vi "Find Supported By.vi"(11 "Bricks in":T1(array[cluster])) -> (3 "Bricks out":T1(array[cluster]))   [LabVIEW 2023, in "d22.lvlib"]
uses:
  d22.lvlib
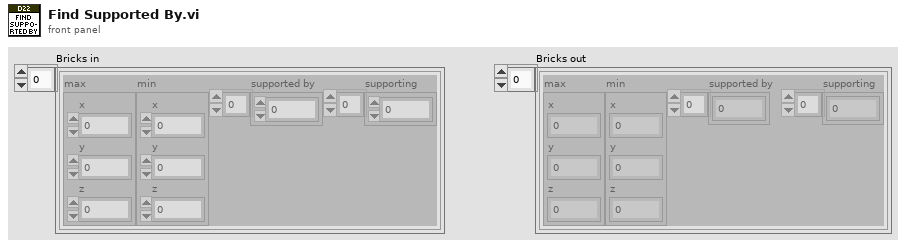
[diagram p1: front panel]
types:
  T1 = cluster{"max":cluster{"x":i32, "y":i32, "z":i32}, "min":cluster{"x":i32, "y":i32, "z":i32}, "supported by":i32[], "supporting":i32[]}[]
  T2 = cluster{"max":cluster{"x":i32, "y":i32, "z":i32}, "min":cluster{"x":i32, "y":i32, "z":i32}, "supported by":i32[], "supporting":i32[]}
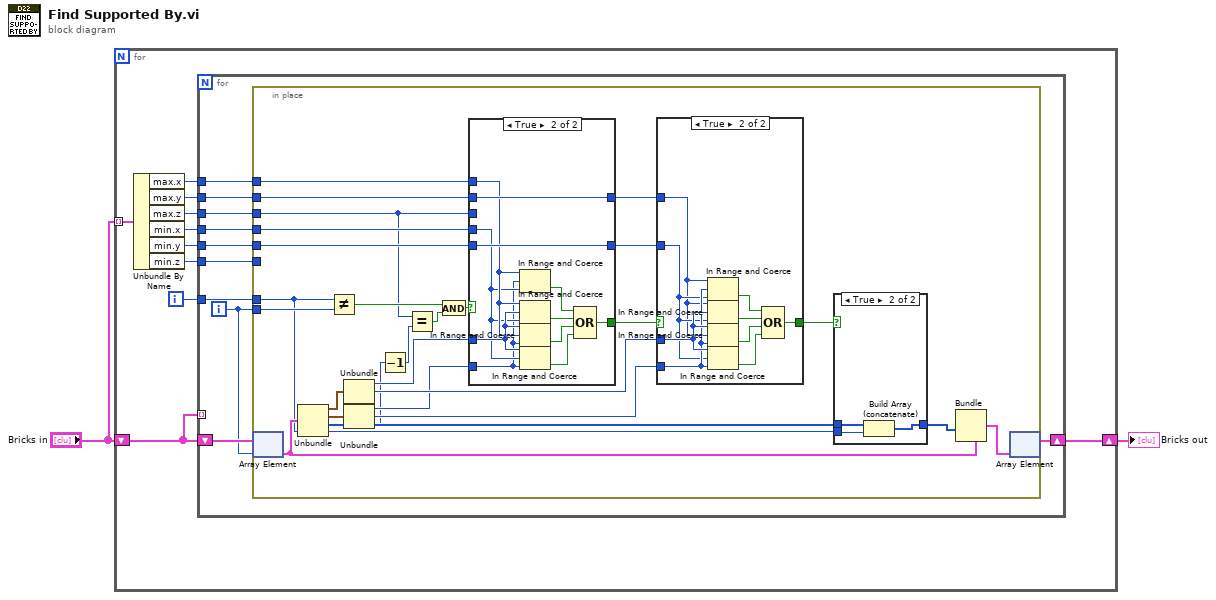
[diagram p0: block diagram]
diagram:
  n1 = for {
    shift-right: [w11] -> w2
    shift-left: "Bricks in" -> [w3]
    tunnel: "Bricks in" -> [w10] mode=indexing
    i -> [w12]
    n2 = Unbundle By Name(w10) -> ("max.x"=w8:i32, "max.y"=w9:i32, "max.z"=w7:i32, "min.x"=w6:i32, "min.y"=w5:i32, "min.z"=w4:i32)
    n3 = for {
      tunnel: w9 -> [w21]
      tunnel: w8 -> [w22]
      tunnel: w7 -> [w20]
      tunnel: w6 -> [w19]
      tunnel: w5 -> [w18]
      tunnel: w4 -> [w17]
      tunnel: w12 -> [w16]
      shift-right: [w13] -> w11
      shift-left: w3 -> [w15]
      tunnel: w3 -> [_] mode=indexing
      i -> [w14]
      n4 = in-place {
        in-place-border: w22 -> [w46]
        in-place-border: w21 -> [w45]
        in-place-border: w20 -> [w24]
        in-place-border: w19 -> [w44]
        in-place-border: w18 -> [w43]
        in-place-border: w17 -> [_]
        in-place-border: w16 -> [w26]
        in-place-border: w14 -> [w31]
        n5 = in-place-array #1(w15, w14) -> (w29:T2)
        n6 = Unbundle(w29) -> ("max"=w48:cluster{"x":i32, "y":i32, "z":i32}, "min"=w47:cluster{"x":i32, "y":i32, "z":i32}, "supported by"=w30:i32[])  [unwired: 1 out]
        n7 = Not Equal?(x=w26, y=w31) -> (x != y?=w37:bool)
        n8 = Unbundle(w48) -> ("x"=w36:i32, "y"=w35:i32)  [unwired: 1 out]
        n9 = Unbundle(w47) -> ("x"=w33:i32, "y"=w34:i32, "z"=w25:i32)
        n10 = Decrement(x=w25) -> (x-1=w23:i32)
        n11 = Equal?(x=w24, y=w23) -> (x = y?=w42:bool)
        n12 = And(x=w37, y=w42) -> (x .and. y?=w38:bool)
        n13 = case shown="True" w38 {
          tunnel: w46 -> [_ w71]
          tunnel: w45 -> [w63 w74]
          tunnel: w24 -> [_ _]
          tunnel: w44 -> [_ w70]
          tunnel: w43 -> [w62 w73]
          tunnel: [_ w64] -> w39
          tunnel: [w63 w74] -> w40
          tunnel: [w62 w73] -> w41
          tunnel: w36 -> [_ w72]
          tunnel: w33 -> [_ w69]
          frame False {
          }
          frame True {
            n14 = In Range and Coerce(upper limit=w71, x=w69, lower limit=w70) -> (In Range?=w65:bool)  [unwired: 1 out]
            n15 = In Range and Coerce(upper limit=w71, x=w72, lower limit=w70) -> (In Range?=w67:bool)  [unwired: 1 out]
            n16 = In Range and Coerce(upper limit=w72, x=w71, lower limit=w69) -> (In Range?=w68:bool)  [unwired: 1 out]
            n17 = In Range and Coerce(upper limit=w72, x=w70, lower limit=w69) -> (In Range?=w66:bool)  [unwired: 1 out]
            n18 = Compound Arithmetic op=OR(w65, w67, w68, w66) -> (w64:bool)
          }
        }
        n19 = case shown="True" w39 {
          tunnel: w40 -> [_ w53]
          tunnel: w41 -> [_ w54]
          tunnel: [_ w55] -> w32
          tunnel: w35 -> [_ w61]
          tunnel: w34 -> [_ w60]
          frame False {
          }
          frame True {
            n20 = In Range and Coerce(upper limit=w53, x=w60, lower limit=w54) -> (In Range?=w56:bool)  [unwired: 1 out]
            n21 = In Range and Coerce(upper limit=w53, x=w61, lower limit=w54) -> (In Range?=w58:bool)  [unwired: 1 out]
            n22 = In Range and Coerce(upper limit=w61, x=w53, lower limit=w60) -> (In Range?=w59:bool)  [unwired: 1 out]
            n23 = In Range and Coerce(upper limit=w61, x=w54, lower limit=w60) -> (In Range?=w57:bool)  [unwired: 1 out]
            n24 = Compound Arithmetic op=OR(w56, w58, w59, w57) -> (w55:bool)
          }
        }
        n25 = case shown="True" w32 {
          tunnel: w30 -> [w49 w52]
          tunnel: [w49 w51] -> w28
          tunnel: w26 -> [_ w50]
          frame False {
          }
          frame True {
            n26 = Build Array (concatenate)(w52, w50) -> (w51:i32[])
          }
        }
        n27 = Bundle(cluster=w29, "supported by"=w28) -> (w27:T2)  [unwired: 3 in]
        n28 = in-place-array #1(w27) -> (w13:T1)  [unwired: 1 out]
      }
    }
  }
  "Bricks out" <- w2
